vi "PLUXmereni.vi"() -> (1 "XY graph visual":cluster{dbl[], dbl[]}(graph))   [LabVIEW 2026]
uses:
  <userlib>/Status.ctl
  <vilib>/Analysis/3filter.llb/Butterworth Filter (DBL).vi
  <vilib>/measure/maspectr.llb/FFT Spectrum (Mag-Phase) for N Chan.vi
  <vilib>/Instr/_visa.llb/VISA Configure Serial Port (Instr).vi
  <vilib>/measure/NI_MAPro.lvlib
  <vilib>/Analysis/NI_AALBase.lvlib
panel:
  out "Array of signals":waveform(dbl)[](array[waveform])
  out "Spectrum":cluster{"f0":dbl, "df":dbl, "magnitude":dbl[]}[](graph)
  in  "EditCluster":T1={"Horní mezní frekvence"=0.45000000000000007, "Dolní mezní frekvence"=0.0, "filter type"=enum."Lowpass", "applyFilter"=FALSE, "removeFilter"=FALSE, "undoFIlter"=FALSE} {"Horní mezní frekvence" format="%0.2f"}
  out "Waveform Graph Edit":waveform(dbl)[](graph)
  out "Zobrazeni typu signalu":cluster{string, string}
  in  "Exit Button":bool
  out "NewVal":bool
  in  "MereniAZpracovaniSwitch":bool
  in  "Cluster":T2={"Zařízení"="", "Cesta k uloženému souboru"=path "", "Vzorkovací frekvence"=enum."1000", "Record Button"=FALSE, "Stop Button"=FALSE, "A1 signál"=enum."EMG", "A2 signál"=enum."EMG", "A3 signál"=enum."EMG", "A4 signál"=enum."EMG", "A5 signál"=enum."EMG", "A6 signál"=enum."EMG", "Pin s připojeným signálem"=enum."A1"}
  in  "DO 4":bool
  in  "DO 3":bool
  in  "DO 2":bool
  in  "DO 1":bool
  out "tdms file":refnum<k34>
  out "Ylabel and Plot name":cluster{string, string}
  out "Sample Rate Numeric":i32
  out "Consumer":i32
  out "producer":i32
  in  "error in (no error)":errorcluster
  out "Sync Stop":bool=TRUE
  # "Aplikace pro měření a zpracování dat na platformě PLUX BITalino"
  # "Spodní tlačítko bude jako switch mez iměřením a zpracováním                     tlačítka filtr, odstranit filtraci, undo"
  # "Hz"
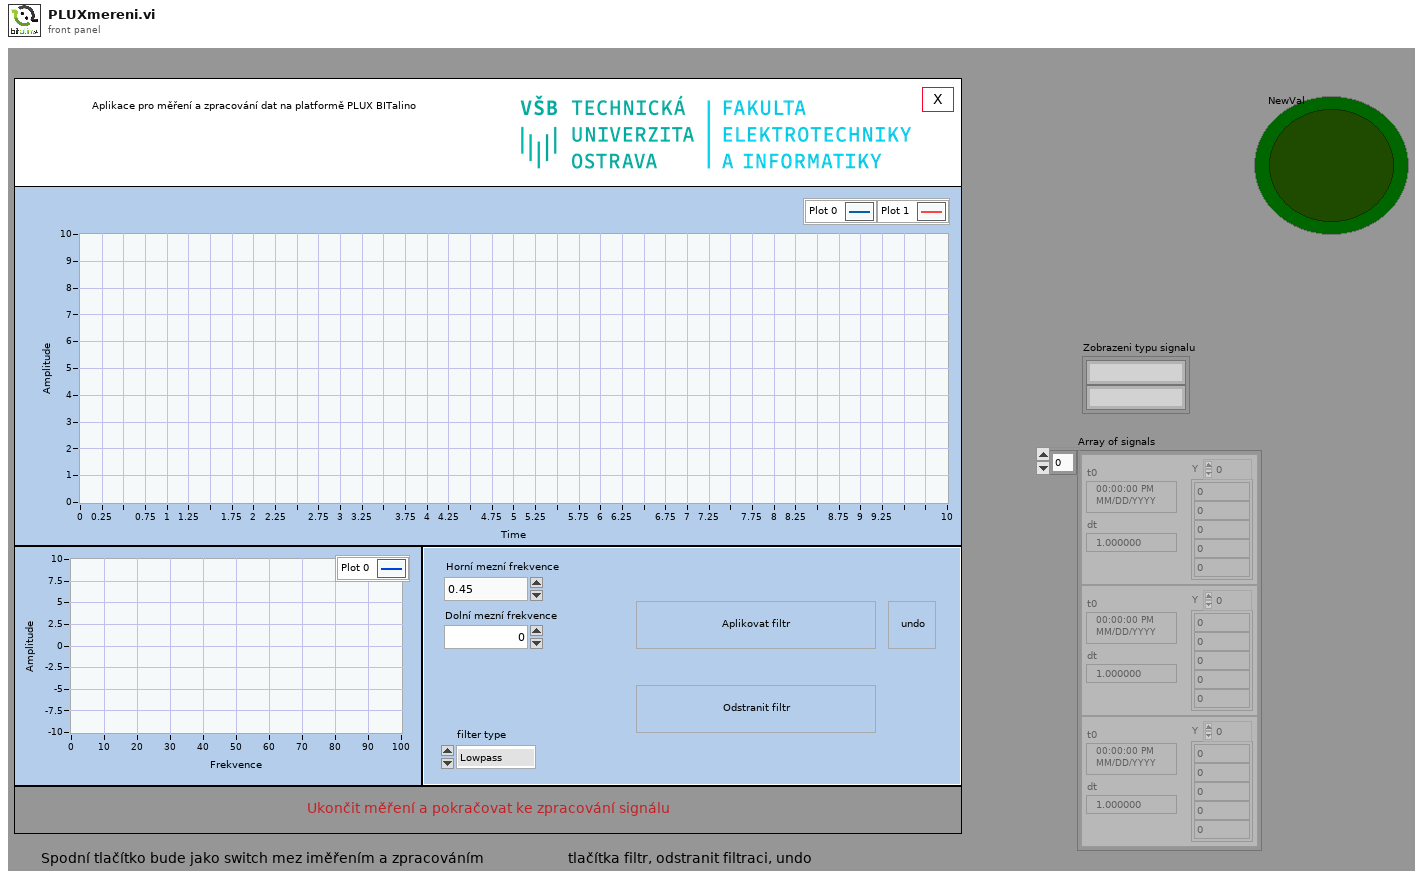
[diagram p1: front panel]
types:
  T1 = cluster{"Horní mezní frekvence":dbl, "Dolní mezní frekvence":dbl, "filter type":enum32{"Lowpass", "Highpass", "Bandpass", "Bandstop"}, "applyFilter":bool, "removeFilter":bool, "undoFIlter":bool}
  T2 = cluster{"Zařízení":refnum<visa-resource-name>, "Cesta k uloženému souboru":path, "Vzorkovací frekvence":enum16{"1", "10", "100", "1000"}, "Record Button":bool, "Stop Button":bool, "A1 signál":enum16{"EMG", "ECG", "EEG", "EDA", "ACC"}, "A2 signál":enum16{"EMG", "ECG", "EEG", "EDA", "ACC"}, "A3 signál":enum16{"EMG", "ECG", "EEG", "EDA", "ACC"}, "A4 signál":enum16{"EMG", "ECG", "EEG", "EDA", "ACC"}, "A5 signál":enum16{"EMG", "ECG", "EEG", "EDA", "ACC"}, "A6 signál":enum16{"EMG", "ECG", "EEG", "EDA", "ACC"}, "Pin s připojeným signálem":enum32{"A1", "A2", "A3", "A4", "A5", "A6"}}
  T3 = enum8{"Enabled", "Disabled", "Disabled and Grayed Out"}
  T4 = enum16{"open", "open or create", "create or replace", "create", "open (read-only)"}
  T5 = typedef "Status.ctl" = enum16{"Initialize", "Edit", "Standby", "Recording", "Exit"}
  T6 = enum32{"Lowpass", "Highpass", "Bandpass", "Bandstop"}
  T7 = cluster{"A1 signál":enum16{"EMG", "ECG", "EEG", "EDA", "ACC"}, "A2 signál":enum16{"EMG", "ECG", "EEG", "EDA", "ACC"}, "A3 signál":enum16{"EMG", "ECG", "EEG", "EDA", "ACC"}, "A4 signál":enum16{"EMG", "ECG", "EEG", "EDA", "ACC"}, "A5 signál":enum16{"EMG", "ECG", "EEG", "EDA", "ACC"}, "A6 signál":enum16{"EMG", "ECG", "EEG", "EDA", "ACC"}}
  T8 = cluster{"Result":dbl, "Result":dbl, "Result":dbl, "Result":dbl, "Result":dbl, "Result":dbl}
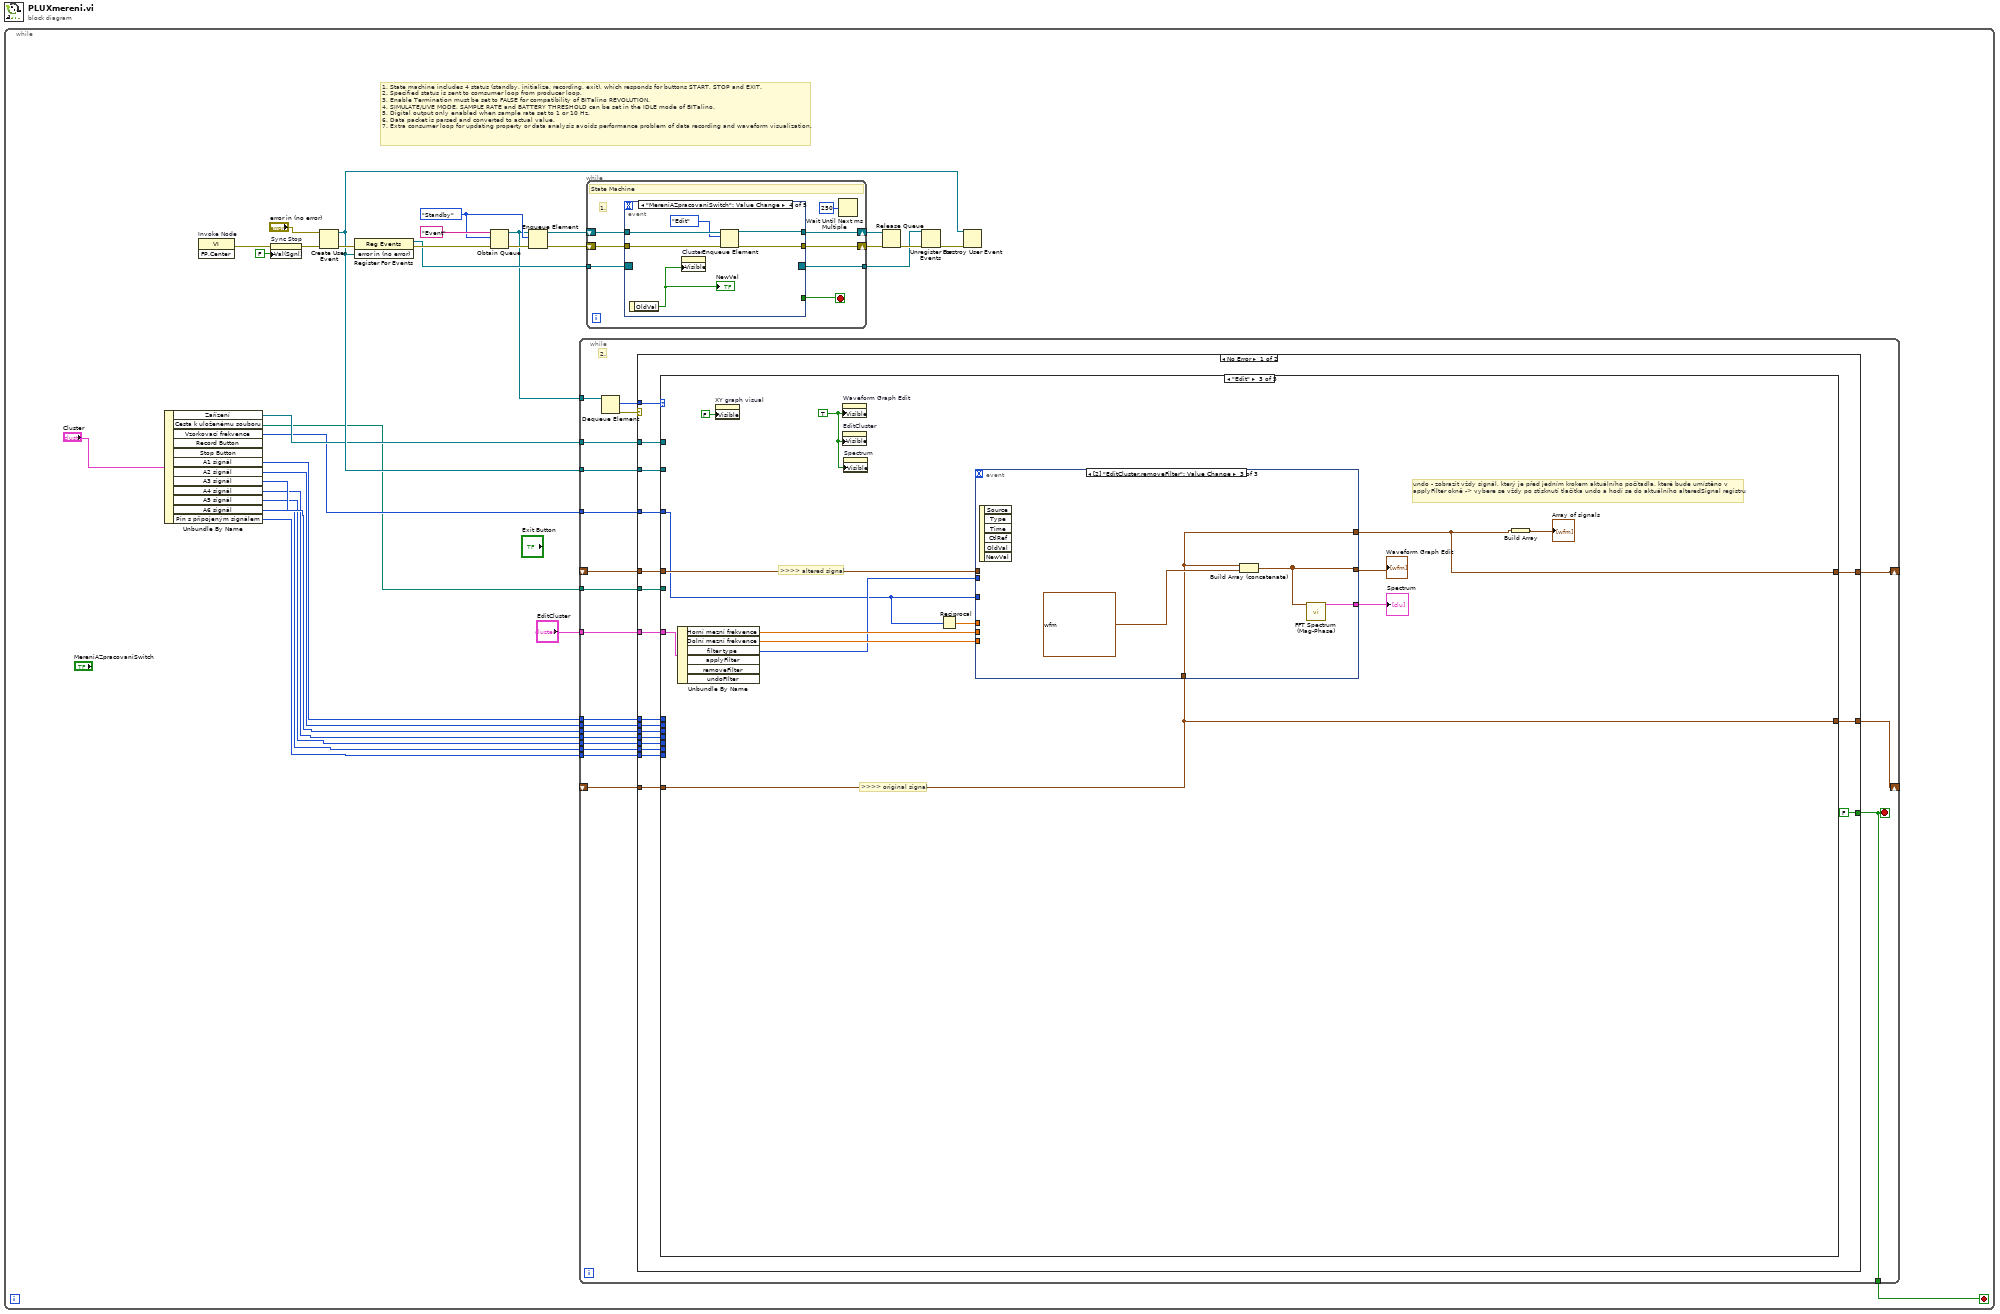
[diagram p0: block diagram]
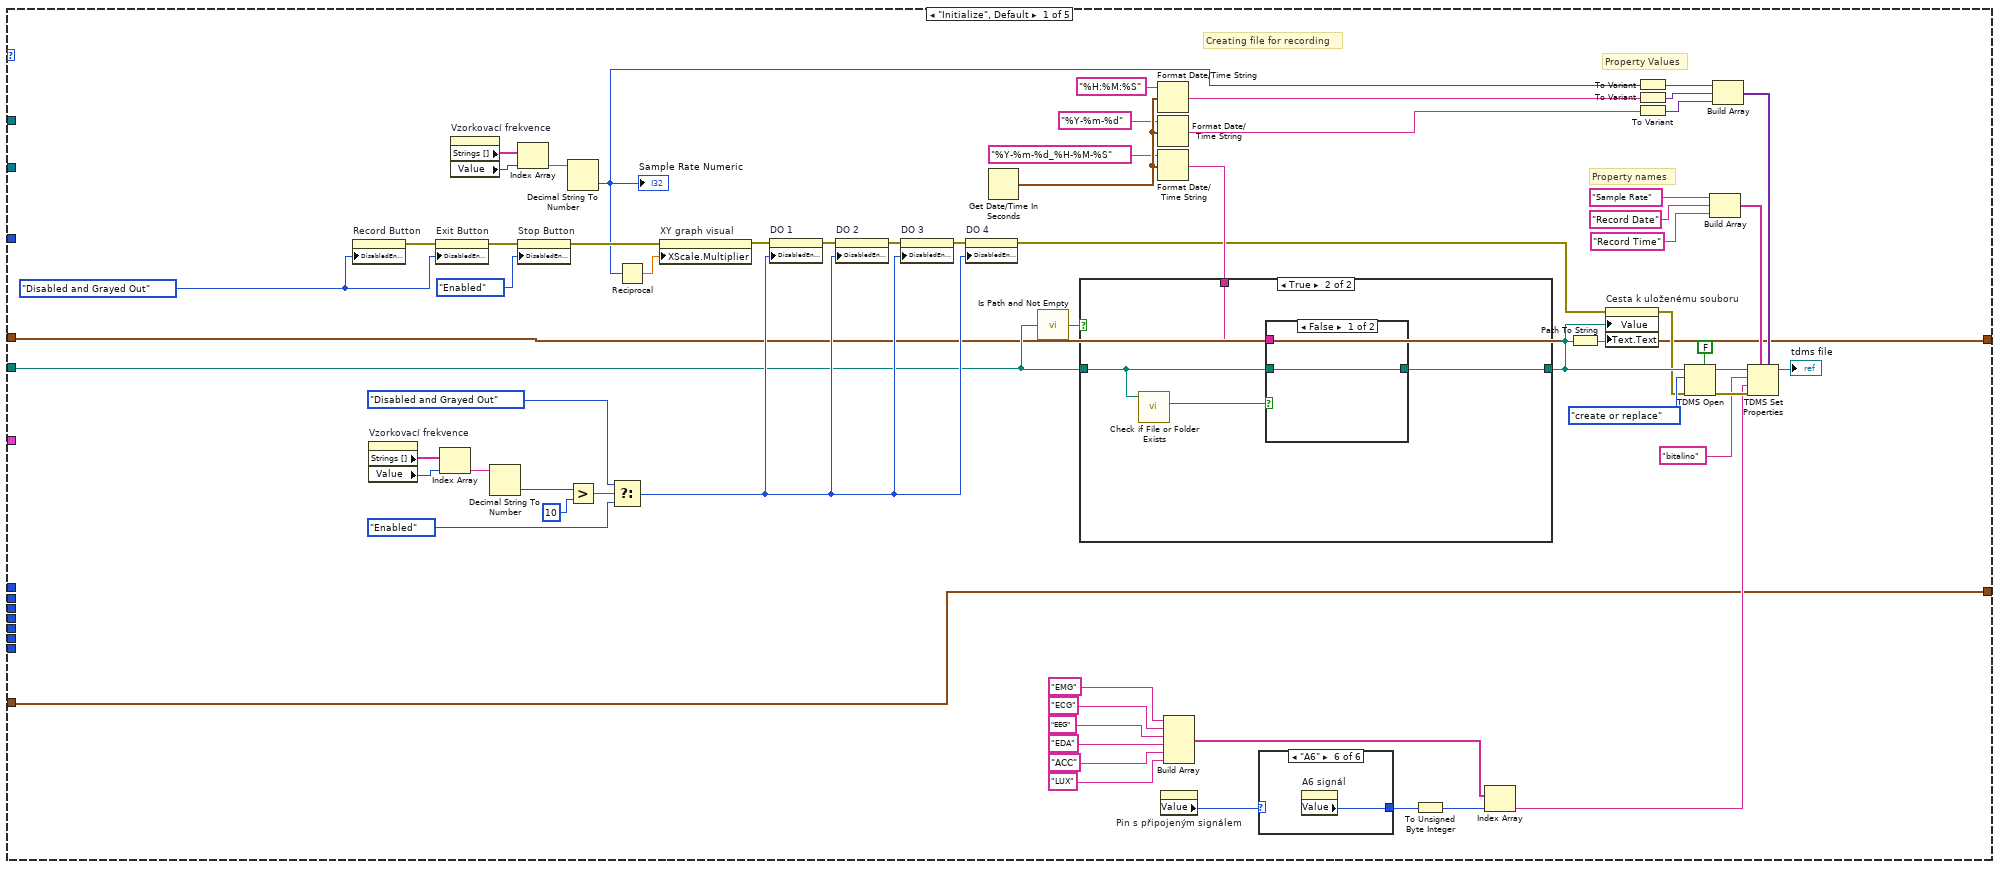
[diagram p2: hidden frame]
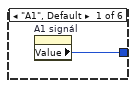
[diagram p3: hidden frame]
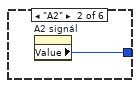
[diagram p4: hidden frame]
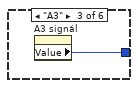
[diagram p5: hidden frame]
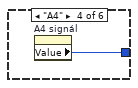
[diagram p6: hidden frame]
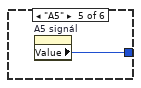
[diagram p7: hidden frame]
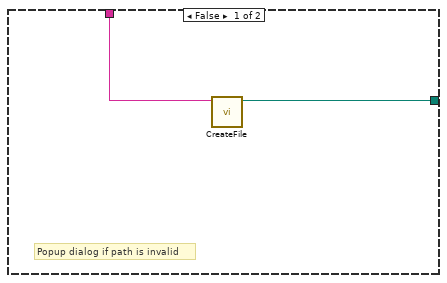
[diagram p8: hidden frame]
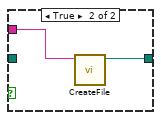
[diagram p9: hidden frame]
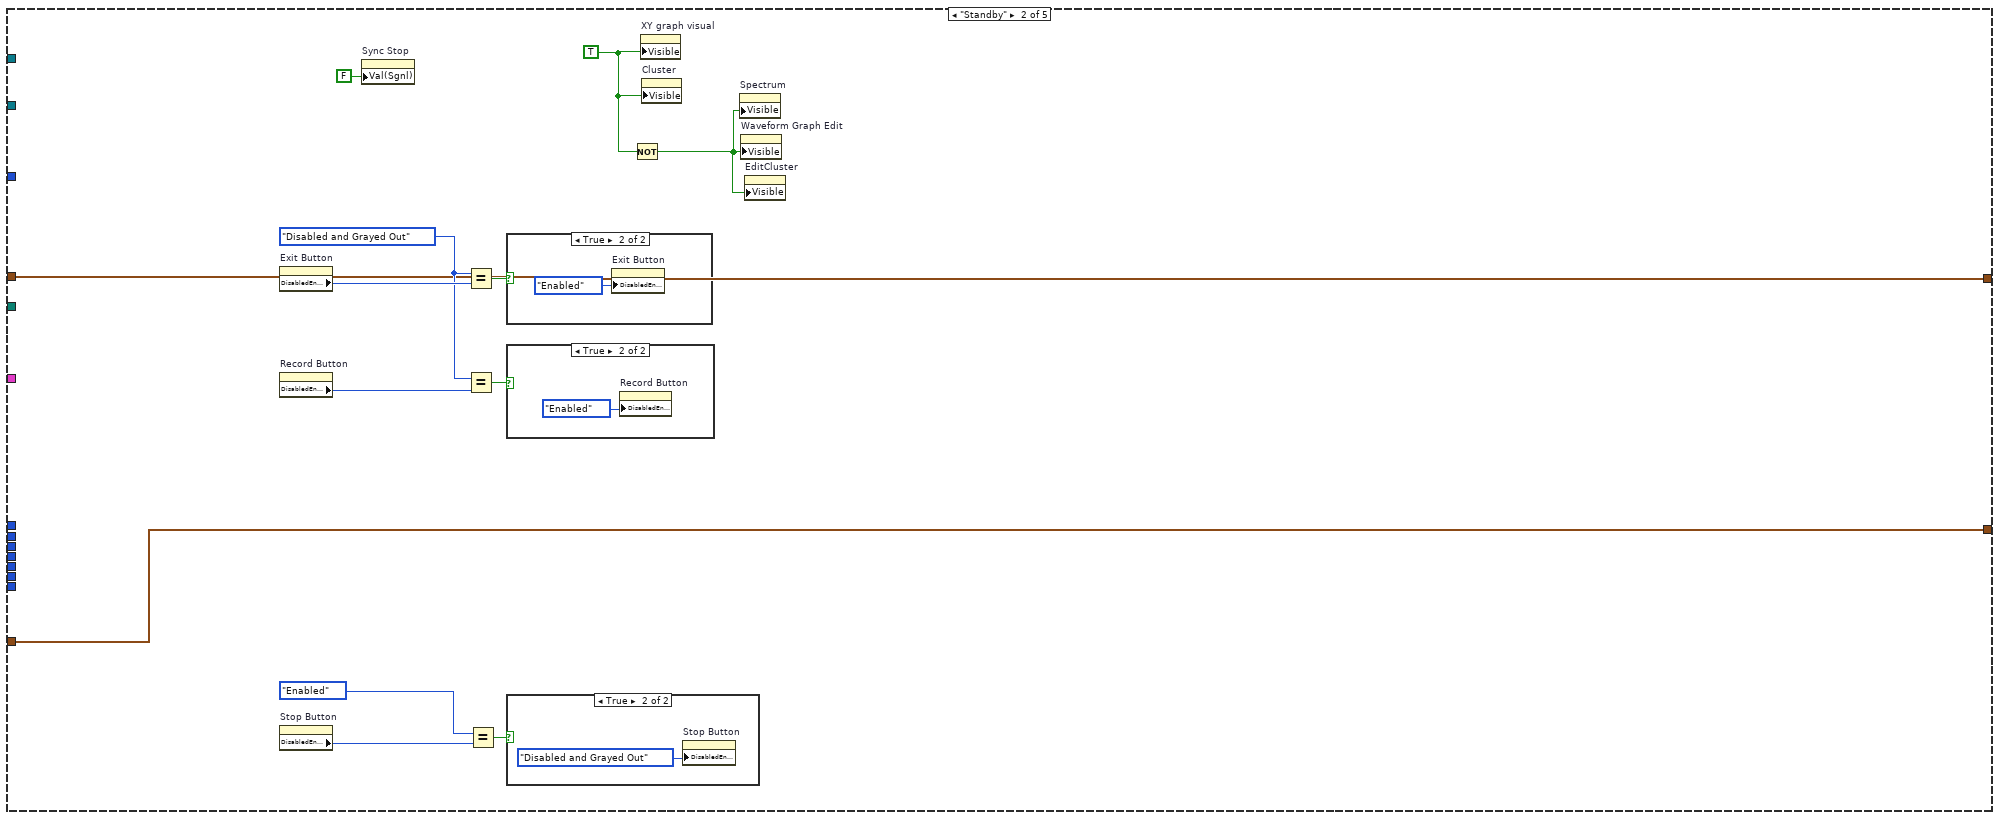
[diagram p10: hidden frame]
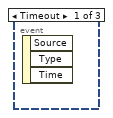
[diagram p14: hidden frame]
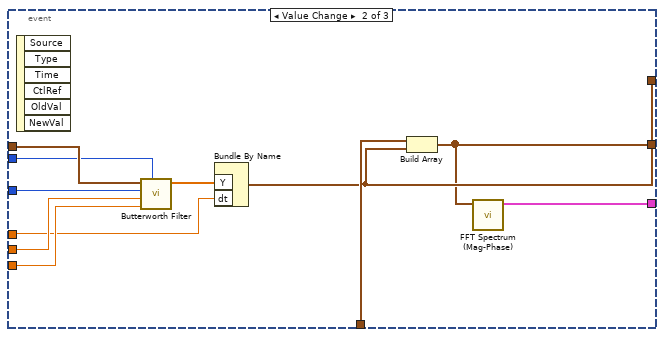
[diagram p15: hidden frame]
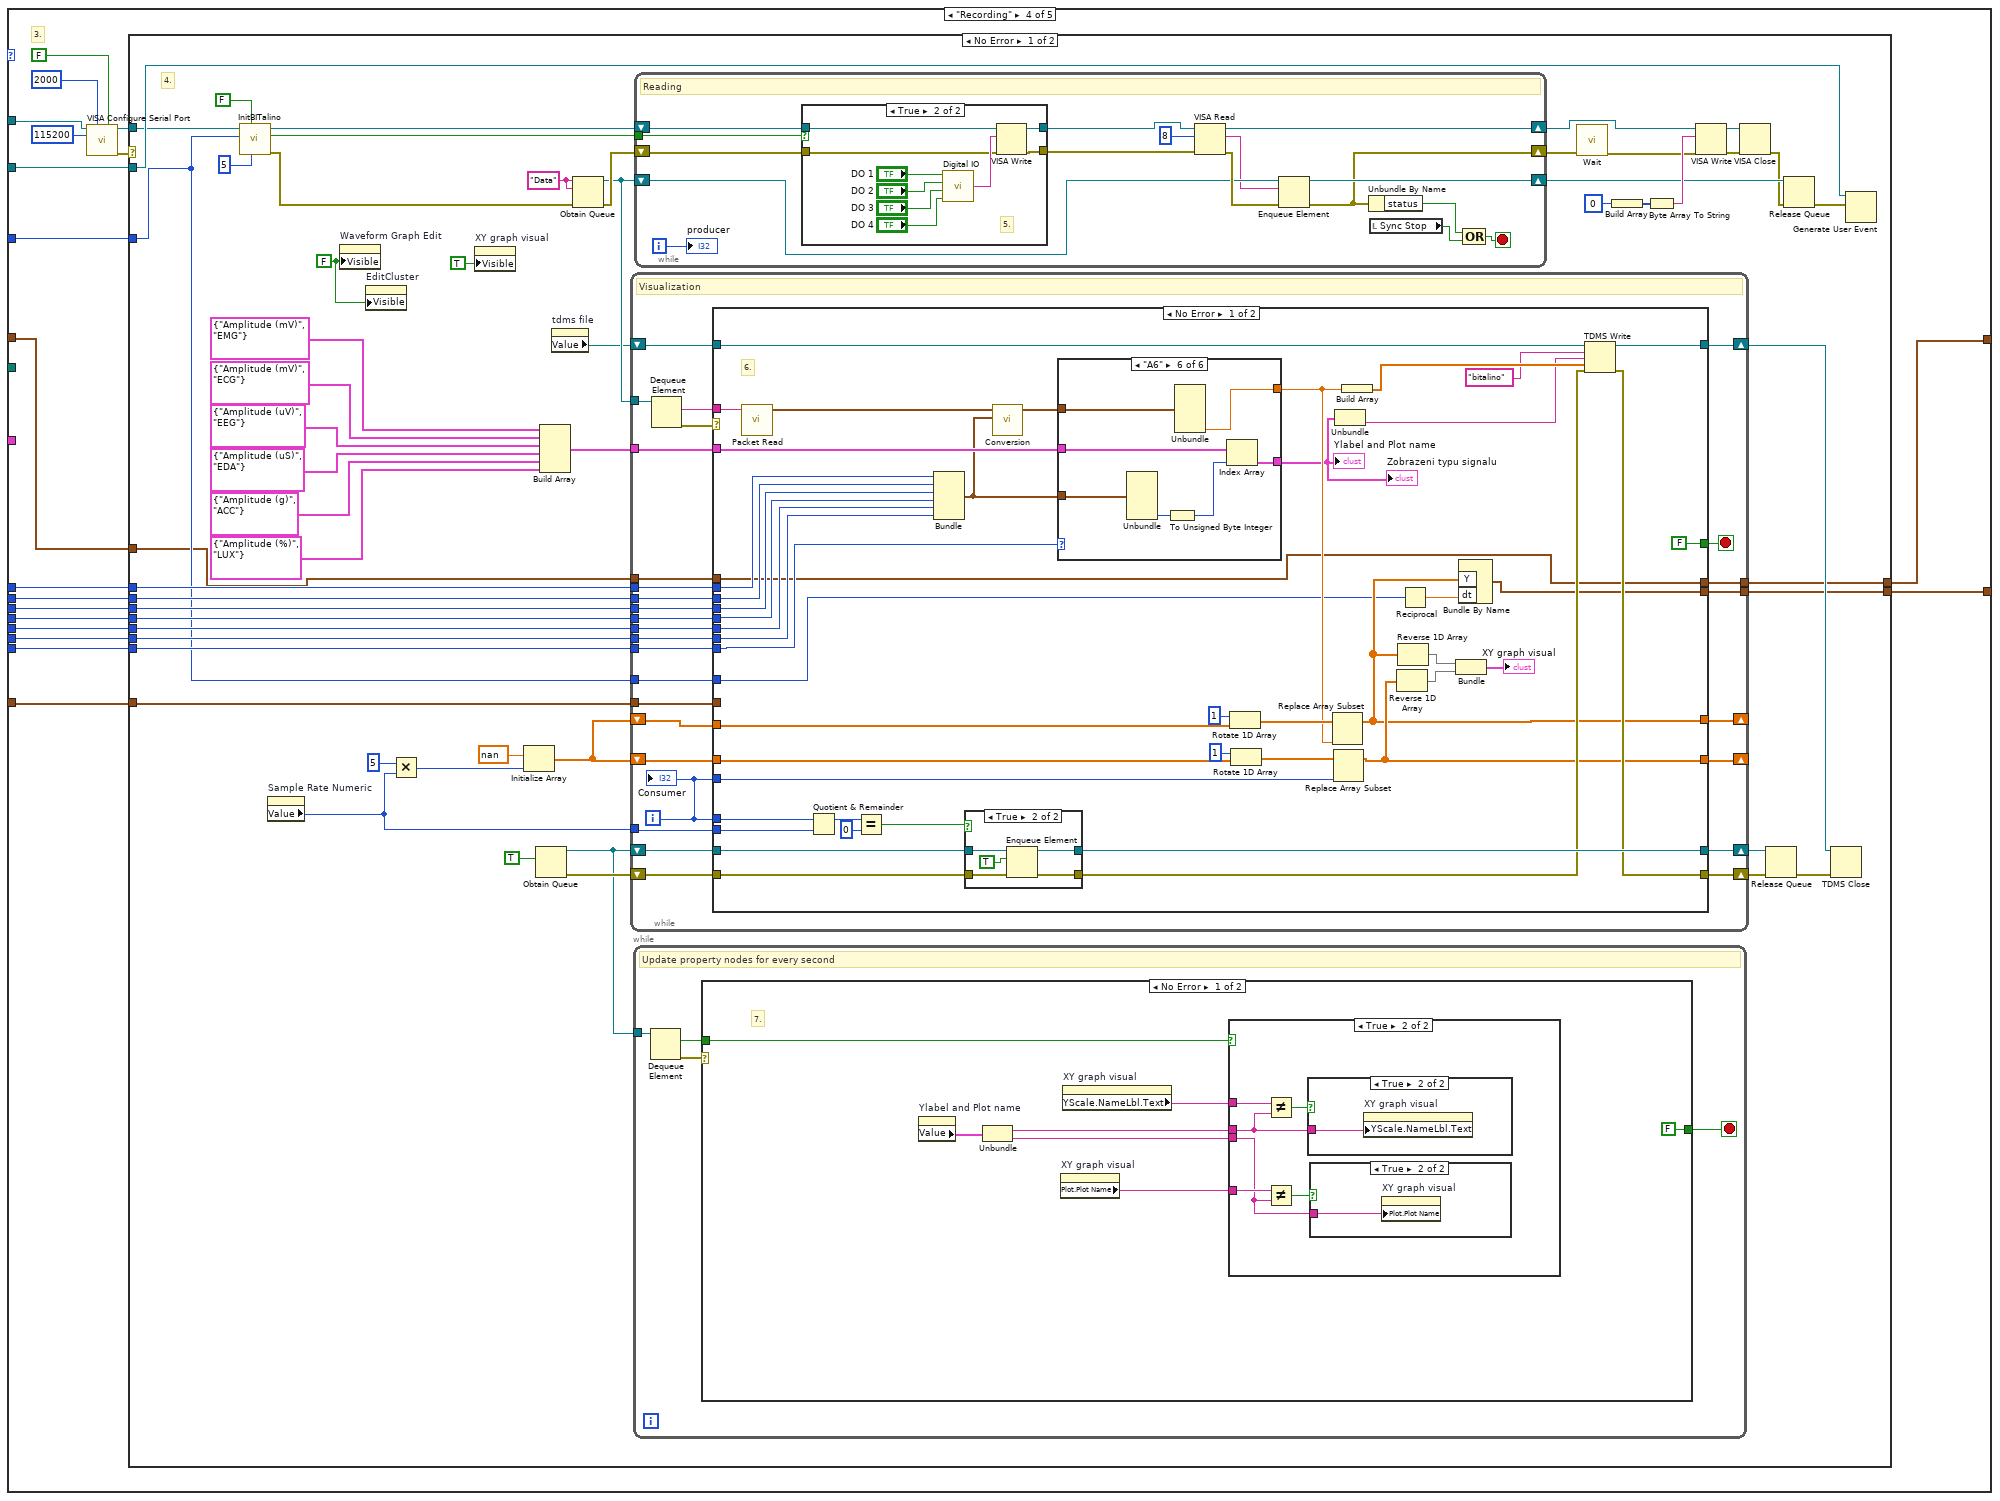
[diagram p16: hidden frame]
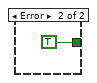
[diagram p20: hidden frame]
diagram:
  n1 = while {
    stop <- w3 stop-if-true
    w31 = Status."Standby" ("Enum")
    # "1. State machine includes 4 status (standby, initialize, recording, exit), which responds for buttons START, STOP and EXIT.\n2. Specified status is sent to comsumer loop from producer loop.\n3. Enable Termination must be set to FALSE for compatibility of BITalino REVOLUTION.\n4. SIMULATE/LIVE MODE, SAMPLE RATE and BATTERY THRESHOLD can be set in the IDLE mode of BITalino.\n5. Digital output only enabled when sample rate set to 1 or 10 Hz.\n6. Data packet is parsed and converted to actual value.\n7. Extra consumer loop for updating property or data analysis avoids performance problem of data recording and waveform visualization."
    n2 = Unbundle By Name("Cluster") -> ("Zařízení"=w13:refnum<visa-resource-name>, "Cesta k uloženému souboru"=w4:path, "Vzorkovací frekvence"=w12:enum16{"1", "10", "100", "1000"}, "A1 signál"=w11:enum16{"EMG", "ECG", "EEG", "EDA", "ACC"}, "A2 signál"=w10:enum16{"EMG", "ECG", "EEG", "EDA", "ACC"}, "A3 signál"=w9:enum16{"EMG", "ECG", "EEG", "EDA", "ACC"}, "A4 signál"=w8:enum16{"EMG", "ECG", "EEG", "EDA", "ACC"}, "A5 signál"=w7:enum16{"EMG", "ECG", "EEG", "EDA", "ACC"}, "A6 signál"=w6:enum16{"EMG", "ECG", "EEG", "EDA", "ACC"}, "Pin s připojeným signálem"=w5:enum32{"A1", "A2", "A3", "A4", "A5", "A6"})  [unwired: 2 out]
    n3 = invoke on="Invoke Node" class="VI" method="FP.Center"() -> (error out=w15:errorcluster)  [unwired: 3 in, 2 out]
    n4 = property on="Sync Stop" class="Bool (strict)"(error in=w15, "Val(Sgnl)"=FALSE ("Value (Signaling)")) -> (error out=w24:errorcluster)  [unwired: 1 in, 1 out]
    n5 = Create User Event(user event datatype="error in (no error)", error in=w24) -> (user event=w16:refnum<user-event>, error out=w23:errorcluster)
    n6 = register-events(error in=w23, w16) -> (reference out=w21:refnum<event-registration>, error out=w22:errorcluster)  [unwired: 1 in]
    n7 = Obtain Queue(name (unnamed)="Event", element data type=w31, error in (no error)=w22) -> (queue out=w14:refnum<queue>, error out=w27:errorcluster)  [unwired: 2 in, 1 out]
    n8 = Enqueue Element(queue=w14, element=w31, error in (no error)=w27) -> (queue out=w25:refnum<queue>, error out=w26:errorcluster)  [unwired: 1 in, 1 out]
    n9 = while {
      tunnel: w14 -> [w52]
      tunnel: w16 -> [w49]
      tunnel: w12 -> [w48]
      tunnel: [w47] -> w3
      tunnel: w13 -> [w46]
      tunnel: w11 -> [w45]
      tunnel: w10 -> [w44]
      tunnel: w9 -> [w43]
      tunnel: w8 -> [w42]
      tunnel: w7 -> [w41]
      tunnel: w6 -> [w40]
      tunnel: w5 -> [w39]
      tunnel: w4 -> [w38]
      shift-right: [w37] -> _
      shift-left: _ -> [w36]
      tunnel: "EditCluster" -> [w35]
      shift-right: [w34] -> _
      shift-left: _ -> [w33]
      stop <- w47 stop-if-true
      # "2."
      n10 = Dequeue Element(queue=w52) -> (element=w51:T5, error out=w50:errorcluster)  [unwired: 2 in, 2 out]
      n11 = case shown="No Error" w50 {
        tunnel: w51 -> [w67 _]
        tunnel: [FALSE TRUE] -> w47
        tunnel: w49 -> [w69 _]
        tunnel: w48 -> [w68 _]
        tunnel: w46 -> [w66 _]
        tunnel: w45 -> [w65 _]
        tunnel: w44 -> [w64 _]
        tunnel: w43 -> [w63 _]
        tunnel: w42 -> [w62 _]
        tunnel: w41 -> [w61 _]
        tunnel: w40 -> [w60 _]
        tunnel: w39 -> [w59 _]
        tunnel: w38 -> [w58 _]
        tunnel: [w57 w456] -> w37
        tunnel: w36 -> [w56 w456]
        tunnel: w35 -> [w55 _]
        tunnel: [w54 w455] -> w34
        tunnel: w33 -> [w53 w455]
        frame No Error {
          n12 = case shown="\"Edit\"" w67 {
            tunnel: w69 -> [_ _ _ w207 _]
            tunnel: w68 -> [_ _ w170 w206 _]
            tunnel: w66 -> [_ _ _ w205 _]
            tunnel: w65 -> [_ _ _ w204 _]
            tunnel: w64 -> [_ _ _ w203 _]
            tunnel: w63 -> [_ _ _ w202 _]
            tunnel: w62 -> [_ _ _ w201 _]
            tunnel: w61 -> [_ _ _ w200 _]
            tunnel: w60 -> [_ _ _ w199 _]
            tunnel: w59 -> [_ _ _ w198 _]
            tunnel: w58 -> [w73 _ _ _ _]
            tunnel: [w72 w152 w167 w197 w452] -> w57
            tunnel: w56 -> [w72 w152 w167 w196 w452]
            tunnel: w55 -> [_ _ w177 _ _]
            tunnel: [w71 w151 w166 w195 w451] -> w54
            tunnel: w53 -> [w71 w151 w175 w194 w451]
            frame "Initialize", Default {
              w101 = T3."Disabled and Grayed Out" ("Disabled")
              # "Creating file for recording"
              # "Property Values"
              # "Property names"
              n13 = property on="Record Button" class="Bool"("DisabledEnum"=w101) -> (error out=w133:errorcluster)  [unwired: 2 in, 1 out]
              n14 = property on="Vzorkovací frekvence" class="Enum (strict)"() -> ("Strings []"=w91:string[], "Value"=w90:enum16{"1", "10", "100", "1000"})  [unwired: 2 in, 2 out]
              n15 = property on="Exit Button" class="Bool"(error in=w133, "DisabledEnum"=w101) -> (error out=w131:errorcluster)  [unwired: 1 in, 1 out]
              n16 = Index Array "Index Array"(array=w91, index=w90) -> (element=w89:string)
              n17 = property on="Vzorkovací frekvence" class="Enum (strict)"() -> ("Strings []"=w130:string[], "Value"=w129:enum16{"1", "10", "100", "1000"})  [unwired: 2 in, 2 out]
              n18 = Decimal String To Number(string=w89) -> (number=w88:i32)  [unwired: 2 in, 1 out]
              n19 = Index Array(array=w130, index=w129) -> (element=w128:string)
              n20 = property on="Stop Button" class="Bool"(error in=w131, "DisabledEnum"=T3."Enabled" ("Disabled")) -> (error out=w127:errorcluster)  [unwired: 1 in, 1 out]
              n21 = Decimal String To Number(string=w128) -> (number=w100:i32)  [unwired: 2 in, 1 out]
              "Sample Rate Numeric" <- w100
              n22 = Greater?(x=w88, y=10) -> (0:w96:bool)
              n23 = Select(t=T3."Disabled and Grayed Out" ("Disabled"), s=w96, f=T3."Enabled" ("Disabled")) -> (s? t:f=w99:T3)
              n24 = Reciprocal(x=w100) -> (1/x=w126:dbl)
              n25 = property on="XY graph visual" class="XYGraph (strict)"(error in=w127, "XScale.Multiplier"=w126) -> (error out=w87:errorcluster)  [unwired: 1 in, 1 out]
              n26 = property on="DO 1" class="Bool (strict)"(error in=w87, "DisabledEnum"=w99) -> (error out=w94:errorcluster)  [unwired: 1 in, 1 out]
              n27 = property on="DO 2" class="Bool (strict)"(error in=w94, "DisabledEnum"=w99) -> (error out=w93:errorcluster)  [unwired: 1 in, 1 out]
              n28 = property on="DO 3" class="Bool (strict)"(error in=w93, "DisabledEnum"=w99) -> (error out=w92:errorcluster)  [unwired: 1 in, 1 out]
              n29 = property on="DO 4" class="Bool (strict)"(error in=w92, "DisabledEnum"=w99) -> (error out=w86:errorcluster)  [unwired: 1 in, 1 out]
              n30 = Get Date/Time In Seconds() -> (seconds since 1Jan1904=w116:timestamp)
              n31 = call <vilib>:"Is Path and Not Empty.vi"("path"=w73) -> ("Is Path and Not Empty?"=w108:bool)  [unwired: 4 in]
              n32 = Format Date/Time String(time format string (%c)="%H:%M:%S", seconds (now)=w116) -> (date/time string=w121:string)  [unwired: 1 in]
              n33 = Format Date/Time String(time format string (%c)="%Y-%m-%d", seconds (now)=w116) -> (date/time string=w122:string)  [unwired: 1 in]
              n34 = Format Date/Time String(time format string (%c)="%Y-%m-%d_%H-%M-%S", seconds (now)=w116) -> (date/time string=w112:string)  [unwired: 1 in]
              n35 = case shown="True" w108 {
                tunnel: [w140 w143] -> w105
                tunnel: w73 -> [_ w142]
                tunnel: w112 -> [w141 w144]
                frame False {
                  # "Popup dialog if path is invalid"
                  n36 = call <userlib>:"CreateFile.vi"("date/time string"=w141) -> ("appended path"=w140:path)  [unwired: 10 in]
                }
                frame True {
                  n37 = call <vilib>:"Check if File or Folder Exists.vi"("path"=w142) -> ("file or folder exists?"=w145:bool)  [unwired: 8 in, 2 out]
                  n38 = case shown="False" w145 {
                    tunnel: w144 -> [_ w148]
                    tunnel: [w146 w147] -> w143
                    tunnel: w142 -> [w146 _]
                    frame False {
                    }
                    frame True {
                      n39 = call <userlib>:"CreateFile.vi"("date/time string"=w148) -> ("appended path"=w147:path)  [unwired: 10 in]
                    }
                  }
                }
              }
              n40 = property on="Pin s připojeným signálem" class="RadioBtnsControl (strict)"() -> ("Value"=w84:enum32{"A1", "A2", "A3", "A4", "A5", "A6"})  [unwired: 2 in, 2 out]
              n41 = Build Array("EMG", "ECG", "EEG", "EDA", "ACC", "LUX") -> (w75:string[])
              n42 = case shown="\"A6\"" w84 {
                tunnel: [w134 w135 w136 w137 w138 w139] -> w77
                frame "A1", Default {
                  n43 = property on="A1 signál" class="Enum (strict)"() -> ("Value"=w134:enum16{"EMG", "ECG", "EEG", "EDA", "ACC"})  [unwired: 2 in, 2 out]
                }
                frame "A2" {
                  n44 = property on="A2 signál" class="Enum (strict)"() -> ("Value"=w135:enum16{"EMG", "ECG", "EEG", "EDA", "ACC"})  [unwired: 2 in, 2 out]
                }
                frame "A3" {
                  n45 = property on="A3 signál" class="Enum (strict)"() -> ("Value"=w136:enum16{"EMG", "ECG", "EEG", "EDA", "ACC"})  [unwired: 2 in, 2 out]
                }
                frame "A4" {
                  n46 = property on="A4 signál" class="Enum (strict)"() -> ("Value"=w137:enum16{"EMG", "ECG", "EEG", "EDA", "ACC"})  [unwired: 2 in, 2 out]
                }
                frame "A5" {
                  n47 = property on="A5 signál" class="Enum (strict)"() -> ("Value"=w138:enum16{"EMG", "ECG", "EEG", "EDA", "ACC"})  [unwired: 2 in, 2 out]
                }
                frame "A6" {
                  n48 = property on="A6 signál" class="Enum (strict)"() -> ("Value"=w139:enum16{"EMG", "ECG", "EEG", "EDA", "ACC"})  [unwired: 2 in, 2 out]
                }
              }
              n49 = To Unsigned Byte Integer(number=w77) -> (unsigned 8bit integer=w76:u8)
              n50 = Index Array(array=w75, index=w76) -> (element=w74:string)
              n51 = Path To String(path=w105) -> (string=w106:string)
              n52 = property on="Cesta k uloženému souboru" class="Path"(error in=w86, "Value"=w105, "Text.Text"=w106) -> (error out=w104:errorcluster)  [unwired: 1 in, 1 out]
              n53 = To Variant(anything=w100) -> (Variant=w120:variant)
              n54 = To Variant(anything=w121) -> (Variant=w123:variant)
              n55 = To Variant(anything=w122) -> (Variant=w124:variant)
              n56 = TDMS Open(5:FALSE ("create index file? (T)"), 8:w104, 10:T4."create or replace" ("operation (0:open)"), 11:w105) -> (0:w111:errorcluster, 3:w110:refnum<k34>)  [unwired: 3 in]
              n57 = Build Array("Sample Rate", "Record Date", "Record Time") -> (w119:string[])
              n58 = Build Array(w120, w123, w124) -> (w125:variant[])
              n59 = TDMS Set Properties(5:w125, 7:w119, 8:w111, 9:w74, 10:"bitalino", 11:w110) -> (3:→"tdms file":refnum<k34>)  [unwired: 3 out]
            }
            frame "Standby" {
              w150 = TRUE ("Visible")
              w153 = T3."Disabled and Grayed Out" ("Disabled")
              n60 = property on="Exit Button" class="Bool"() -> ("DisabledEnum"=w160:T3)  [unwired: 2 in, 2 out]
              n61 = property on="Record Button" class="Bool"() -> ("DisabledEnum"=w158:T3)  [unwired: 2 in, 2 out]
              n62 = property on="Stop Button" class="Bool"() -> ("DisabledEnum"=w155:T3)  [unwired: 2 in, 2 out]
              n63 = property on="Sync Stop" class="Bool (strict)"("Val(Sgnl)"=FALSE ("Value (Signaling)")) -> ()  [unwired: 2 in, 2 out]
              n64 = Equal?(x=w153, y=w160) -> (x = y?=w159:bool)
              n65 = Equal?(x=w153, y=w158) -> (x = y?=w157:bool)
              n66 = Equal?(x=T3."Enabled" ("Disabled"), y=w155) -> (x = y?=w154:bool)
              n67 = case shown="True" w159 {
                frame False {
                }
                frame True {
                  n68 = property on="Exit Button" class="Bool"("DisabledEnum"=T3."Enabled" ("Disabled")) -> ()  [unwired: 2 in, 2 out]
                }
              }
              n69 = case shown="True" w157 {
                frame False {
                }
                frame True {
                  n70 = property on="Record Button" class="Bool"("DisabledEnum"=T3."Enabled" ("Disabled")) -> ()  [unwired: 2 in, 2 out]
                }
              }
              n71 = case shown="True" w154 {
                frame False {
                }
                frame True {
                  n72 = property on="Stop Button" class="Bool"("DisabledEnum"=T3."Disabled and Grayed Out" ("Disabled")) -> ()  [unwired: 2 in, 2 out]
                }
              }
              n73 = Not(x=w150) -> (.not. x?=w149:bool)
              n74 = property on="XY graph visual" class="XYGraph (strict)"("Visible"=w150) -> ()  [unwired: 2 in, 2 out]
              n75 = property on="Cluster" class="Clust"("Visible"=w150) -> ()  [unwired: 2 in, 2 out]
              n76 = property on="Spectrum" class="WFGraph (strict)"("Visible"=w149) -> ()  [unwired: 2 in, 2 out]
              n77 = property on="Waveform Graph Edit" class="WFGraph (strict)"("Visible"=w149) -> ()  [unwired: 2 in, 2 out]
              n78 = property on="EditCluster" class="Clust"("Visible"=w149) -> ()  [unwired: 2 in, 2 out]
            }
            frame "Edit" {
              w176 = TRUE ("Visible")
              # "undo - zobrazit vždy signál, který je před jedním krokem aktuálního počítadla, které bude umístěno v \napplyFilter okně -> vybere se vždy po stisknutí tlačítka undo a hodí se do aktuálního alteredSignal registru"
              # ">>>> altered signal"
              # ">>>> original signal"
              n79 = Unbundle By Name(w177) -> ("Horní mezní frekvence"=w173:dbl, "Dolní mezní frekvence"=w172:dbl, "filter type"=w171:T6)  [unwired: 3 out]
              n80 = property on="XY graph visual" class="XYGraph (strict)"("Visible"=FALSE) -> ()  [unwired: 2 in, 2 out]
              n81 = property on="Waveform Graph Edit" class="WFGraph (strict)"("Visible"=w176) -> ()  [unwired: 2 in, 2 out]
              n82 = property on="EditCluster" class="Clust"("Visible"=w176) -> ()  [unwired: 2 in, 2 out]
              n83 = property on="Spectrum" class="WFGraph (strict)"("Visible"=w176) -> ()  [unwired: 2 in, 2 out]
              n84 = Reciprocal(x=w170) -> (1/x=w174:dbl)
              n85 = event shown="[2] \"EditCluster.removeFilter\": Value Change" {
                selector: _ -> [_ _ _]
                dyn-events: _ -> [_ _ _]
                timeout: _ -> [_ _ _]
                tunnel: w167 -> [_ w188 w190]
                tunnel: [_ w187 w190] -> w166
                tunnel: w175 -> [_ w186 _]
                tunnel: w174 -> [_ w182 _]
                tunnel: w173 -> [_ w185 _]
                tunnel: w172 -> [_ w184 _]
                tunnel: w171 -> [_ w183 _]
                tunnel: w170 -> [_ w181 _]
                tunnel: [_ w180 w191] -> w169
                tunnel: [_ w179 w192] -> w168
                event Timeout {
                  n86 = event-data() -> ()  [unwired: 1 in, 3 out]
                }
                event "EditCluster.applyFilter": Value Change {
                  n87 = event-data() -> ()  [unwired: 1 in, 6 out]
                  n88 = call-poly <vilib>:"Butterworth Filter.vi"("filter type"=w183, "low cutoff freq: fl"=w184, "high cutoff freq: fh"=w185, "sampling freq: fs"=w181, "X"=w186) -> ("Filtered X"=w189:dbl[])  [unwired: 3 in, 1 out]
                  n89 = Bundle By Name("Y"=w189, "dt"=w182) -> (w187:waveform(dbl))  [unwired: 1 in]
                  n90 = Build Array(w188, w187) -> (w180:waveform(dbl)[])
                  n91 = call-poly <vilib>:"FFT Spectrum (Mag-Phase).vi"("time signals"=w180) -> ("magnitudes"=w179:cluster{"f0":dbl, "df":dbl, "magnitude":dbl[]}[])  [unwired: 6 in, 4 out]
                }
                event "EditCluster.removeFilter": Value Change {
                  n92 = event-data() -> ()  [unwired: 1 in, 6 out]
                  n93 = Build Array (concatenate)(w190, waveform(dbl)[] [{"t0"=timestamp(-3600 s since 1904-01-01), "dt"=0.0, "Y"=[0.0]}] ("array")) -> (w191:waveform(dbl)[])
                  n94 = call-poly <vilib>:"FFT Spectrum (Mag-Phase).vi"("time signals"=w191) -> ("magnitudes"=w192:cluster{"f0":dbl, "df":dbl, "magnitude":dbl[]}[])  [unwired: 6 in, 4 out]
                }
              }
              "Waveform Graph Edit" <- w169
              "Spectrum" <- w168
              n95 = Build Array(w166) -> (→"Array of signals":waveform(dbl)[])
            }
            frame "Recording" {
              # "3."
              n96 = call-poly "VISA Configure Serial Port"("VISA resource name"=w205, "timeout (10sec)"=u32 2000, "Enable Termination\nChar (T)"=FALSE ("Enable Termination\nChar (T)"), "baud rate (9600)"=u32 115200) -> ("VISA resource name out"=w210:refnum<visa-resource-name>, "error out"=w209:errorcluster)  [unwired: 10 in]
              n97 = case shown="No Error" w209 {
                selector: w209 -> [_ w449]
                tunnel: w210 -> [w252 _]
                tunnel: w207 -> [w254 w450]
                tunnel: w206 -> [w219 _]
                tunnel: w204 -> [w228 _]
                tunnel: w203 -> [w227 _]
                tunnel: w202 -> [w226 _]
                tunnel: w201 -> [w225 _]
                tunnel: w200 -> [w224 _]
                tunnel: w199 -> [w223 _]
                tunnel: w198 -> [w222 _]
                tunnel: [w218 w448] -> w197
                tunnel: w196 -> [w216 w448]
                tunnel: [w215 w447] -> w195
                tunnel: w194 -> [w214 w447]
                frame No Error {
                  w213 = FALSE ("Visible")
                  w262 = "Data"
                  # "4."
                  n98 = call <userlib>:"InitBITalino.vi"("Battery \nThreshold (%)"=u8 5 ("Battery \nThreshold (%)"), "MODE"=FALSE, "Sample Rate"=w219, "BITalino"=w252) -> ("error out"=w230:errorcluster, "Digital Output"=w231:bool, "VISA out"=w232:refnum<visa-resource-name>)  [unwired: 5 in]
                  n99 = property on="Sample Rate Numeric" class="DigNum (strict)"() -> ("Value"=w246:i32)  [unwired: 2 in, 2 out]
                  n100 = property on="Waveform Graph Edit" class="WFGraph (strict)"("Visible"=w213) -> ()  [unwired: 2 in, 2 out]
                  n101 = property on="EditCluster" class="Clust"("Visible"=w213) -> ()  [unwired: 2 in, 2 out]
                  n102 = Multiply(x=5, y=w246) -> (x*y=w244:i32)
                  n103 = property on="XY graph visual" class="XYGraph (strict)"("Visible"=TRUE) -> ()  [unwired: 2 in, 2 out]
                  n104 = Initialize Array(nan ("element"), w244) -> (w243:dbl[])
                  n105 = Obtain Queue(element data type=TRUE) -> (queue out=w249:refnum<queue>, error out=w251:errorcluster)  [unwired: 4 in, 1 out]
                  n106 = Build Array(cluster{string, string} {"Amplitude (mV)", "EMG"}, cluster{string, string} {"Amplitude (mV)", "ECG"}, cluster{string, string} {"Amplitude (uV)", "EEG"}, cluster{string, string} {"Amplitude (uS)", "EDA"}, cluster{string, string} {"Amplitude (g)", "ACC"}, cluster{string, string} {"Amplitude (%)", "LUX"}) -> (w236:cluster{string, string}[])
                  n107 = property on="tdms file" class="Ref (strict)"() -> ("Value"=w235:refnum<k34>)  [unwired: 2 in, 2 out]
                  n108 = Obtain Queue(name (unnamed)=w262, element data type=w262, error in (no error)=w230) -> (queue out=w263:refnum<queue>, error out=w264:errorcluster)  [unwired: 2 in, 1 out]
                  n109 = while {
                    tunnel: w263 -> [w316]
                    shift-right: [w311] -> _
                    shift-left: w243 -> [w312]
                    tunnel: w246 -> [w310]
                    shift-right: [w307] -> w248
                    shift-left: w249 -> [w309]
                    shift-right: [w306] -> w247
                    shift-left: w251 -> [w308]
                    shift-right: [w303] -> _
                    shift-left: w243 -> [w305]
                    tunnel: w236 -> [w302]
                    shift-right: [w300] -> w233
                    shift-left: w235 -> [w301]
                    tunnel: w228 -> [w299]
                    tunnel: w227 -> [w298]
                    tunnel: w226 -> [w297]
                    tunnel: w225 -> [w296]
                    tunnel: w224 -> [w295]
                    tunnel: w223 -> [w294]
                    tunnel: w222 -> [w293]
                    tunnel: w219 -> [w292]
                    tunnel: [w291] -> w218
                    tunnel: w216 -> [w290]
                    tunnel: [w289] -> w215
                    tunnel: w214 -> [w288]
                    i -> [w304]
                    stop <- w314 stop-if-true
                    # "Visualization"
                    n110 = Dequeue Element(queue=w316) -> (element=w313:string, error out=w315:errorcluster)  [unwired: 2 in, 2 out]
                    n111 = case shown="No Error" w315 {
                      tunnel: [FALSE TRUE] -> w314
                      tunnel: w313 -> [w337 _]
                      tunnel: w312 -> [w350 w418]
                      tunnel: [w321 w418] -> w311
                      tunnel: w310 -> [w351 _]
                      tunnel: w304 -> [w356 _]
                      tunnel: w309 -> [w359 w417]
                      tunnel: w308 -> [w358 w416]
                      tunnel: [w357 w417] -> w307
                      tunnel: [w338 w416] -> w306
                      tunnel: w305 -> [w347 w415]
                      tunnel: w304 -> [w346 _]
                      tunnel: [w326 w415] -> w303
                      tunnel: w302 -> [w345 _]
                      tunnel: w301 -> [w343 w414]
                      tunnel: [w342 w414] -> w300
                      tunnel: w299 -> [w333 _]
                      tunnel: w298 -> [w332 _]
                      tunnel: w297 -> [w331 _]
                      tunnel: w296 -> [w330 _]
                      tunnel: w295 -> [w329 _]
                      tunnel: w294 -> [w328 _]
                      tunnel: w293 -> [w327 _]
                      tunnel: w292 -> [w319 _]
                      tunnel: [w318 w413] -> w291
                      tunnel: w290 -> [_ w413]
                      tunnel: [w317 w412] -> w289
                      tunnel: w288 -> [w317 w412]
                      frame No Error {
                        # "6."
                        n112 = call <userlib>:"Packet Read.vi"("Packets"=w337) -> ("Analog Channels"=w336:cluster{u16, u16, u16, u16, u16, u16})  [unwired: 7 in, 3 out]
                        n113 = Quotient & Remainder(x=w356, y=w351) -> (x-y*floor(x/y)=w355:i32)  [unwired: 1 out]
                        n114 = Equal?(x=w355, y=0) -> (x = y?=w353:bool)
                        n115 = Bundle "Bundle"("A1 signál"=w333, "A2 signál"=w332, "A3 signál"=w331, "A4 signál"=w330, "A5 signál"=w329, "A6 signál"=w328) -> (w344:T7)  [unwired: 1 in]
                        n116 = case shown="True" w353 {
                          tunnel: w359 -> [w364 w369]
                          tunnel: w358 -> [w363 w368]
                          tunnel: [w364 w367] -> w357
                          tunnel: [w363 w366] -> w341
                          frame False {
                          }
                          frame True {
                            n117 = Enqueue Element(queue=w369, element=TRUE, error in (no error)=w368) -> (queue out=w367:refnum<queue>, error out=w366:errorcluster)  [unwired: 1 in, 1 out]
                          }
                        }
                        n118 = call <userlib>:"Conversion.vi"("Sensor Type"=w344, "Analog Channels"=w336) -> ("Converted Values"=w361:T8)  [unwired: 8 in, 1 out]
                        n119 = case shown="\"A6\"" w327 {
                          tunnel: w361 -> [w376 w383 w390 w397 w404 w411]
                          tunnel: [w375 w382 w389 w396 w403 w410] -> w340
                          tunnel: w345 -> [w371 w378 w385 w393 w399 w407]
                          tunnel: w344 -> [w374 w380 w387 w394 w401 w408]
                          tunnel: [w370 w377 w386 w392 w400 w406] -> w323
                          frame "A1", Default {
                            n120 = Unbundle(w374) -> ("A1 signál"=w372:enum16{"EMG", "ECG", "EEG", "EDA", "ACC"})  [unwired: 5 out]
                            n121 = To Unsigned Byte Integer(number=w372) -> (unsigned 8bit integer=w373:u8)
                            n122 = Unbundle(w376) -> ("Result"=w375:dbl)  [unwired: 5 out]
                            n123 = Index Array(array=w371, index=w373) -> (element=w370:cluster{string, string})
                          }
                          frame "A2" {
                            n124 = Unbundle(w380) -> ("A2 signál"=w379:enum16{"EMG", "ECG", "EEG", "EDA", "ACC"})  [unwired: 5 out]
                            n125 = To Unsigned Byte Integer(number=w379) -> (unsigned 8bit integer=w381:u8)
                            n126 = Unbundle(w383) -> ("Result"=w382:dbl)  [unwired: 5 out]
                            n127 = Index Array(array=w378, index=w381) -> (element=w377:cluster{string, string})
                          }
                          frame "A3" {
                            n128 = Unbundle(w387) -> ("A3 signál"=w384:enum16{"EMG", "ECG", "EEG", "EDA", "ACC"})  [unwired: 5 out]
                            n129 = To Unsigned Byte Integer(number=w384) -> (unsigned 8bit integer=w388:u8)
                            n130 = Unbundle(w390) -> ("Result"=w389:dbl)  [unwired: 5 out]
                            n131 = Index Array(array=w385, index=w388) -> (element=w386:cluster{string, string})
                          }
                          frame "A4" {
                            n132 = Unbundle(w394) -> ("A4 signál"=w391:enum16{"EMG", "ECG", "EEG", "EDA", "ACC"})  [unwired: 5 out]
                            n133 = To Unsigned Byte Integer(number=w391) -> (unsigned 8bit integer=w395:u8)
                            n134 = Unbundle(w397) -> ("Result"=w396:dbl)  [unwired: 5 out]
                            n135 = Index Array(array=w393, index=w395) -> (element=w392:cluster{string, string})
                          }
                          frame "A5" {
                            n136 = Unbundle(w401) -> ("A5 signál"=w398:enum16{"EMG", "ECG", "EEG", "EDA", "ACC"})  [unwired: 5 out]
                            n137 = Unbundle(w404) -> ("Result"=w403:dbl)  [unwired: 5 out]
                            n138 = To Unsigned Byte Integer(number=w398) -> (unsigned 8bit integer=w402:u8)
                            n139 = Index Array(array=w399, index=w402) -> (element=w400:cluster{string, string})
                          }
                          frame "A6" {
                            n140 = Unbundle(w408) -> ("A6 signál"=w405:enum16{"EMG", "ECG", "EEG", "EDA", "ACC"})  [unwired: 5 out]
                            n141 = To Unsigned Byte Integer(number=w405) -> (unsigned 8bit integer=w409:u8)
                            n142 = Unbundle(w411) -> ("Result"=w410:dbl)  [unwired: 5 out]
                            n143 = Index Array(array=w407, index=w409) -> (element=w406:cluster{string, string})
                          }
                        }
                        "Ylabel and Plot name" <- w323
                        "Zobrazeni typu signalu" <- w323
                        n144 = Rotate 1D Array(1:w350, 2:1 ("n")) -> (0:w352:dbl[])
                        n145 = Rotate 1D Array(1:w347, 2:1 ("n")) -> (0:w348:dbl[])
                        n146 = Replace Array Subset(array=w352, new element=w340) -> (w321:dbl[])  [unwired: 1 in]
                        n147 = Replace Array Subset(array=w348, new element=w346) -> (w326:dbl[])  [unwired: 1 in]
                        n148 = Unbundle(w323) -> (w335:string)  [unwired: 1 out]
                        n149 = Build Array(w340) -> (w339:dbl[])
                        n150 = Reverse 1D Array(array=w326) -> (reversed array=w325:dbl[])
                        n151 = Reverse 1D Array(array=w321) -> (reversed array=w322:dbl[])
                        n152 = Reciprocal(x=w319) -> (1/x=w320:dbl)
                        n153 = Bundle(w322, w325) -> (→"XY graph visual":cluster{dbl[], dbl[]})  [unwired: 1 in]
                        n154 = Bundle By Name("Y"=w321, "dt"=w320) -> (w318:waveform(dbl))  [unwired: 1 in]
                        n155 = TDMS Write(0:w343, 5:"bitalino", 7:w335, 9:w339, 11:w341) -> (4:w342:refnum<k34>, 15:w338:errorcluster)  [unwired: 1 in, 2 out]
                      }
                      frame Error {
                      }
                    }
                    "Consumer" <- w304
                  }
                  n156 = while {
                    tunnel: w249 -> [w271]
                    stop <- w268 stop-if-true
                    # "Update property nodes for every second"
                    n157 = Dequeue Element(queue=w271) -> (element=w269:bool, error out=w270:errorcluster)  [unwired: 2 in, 2 out]
                    n158 = case shown="No Error" w270 {
                      tunnel: w269 -> [w275 _]
                      tunnel: [FALSE TRUE] -> w268
                      frame No Error {
                        # "7."
                        n159 = property on="Ylabel and Plot name" class="Clust (strict)"() -> ("Value"=w278:cluster{string, string})  [unwired: 2 in, 2 out]
                        n160 = Unbundle(w278) -> (w277:string, w276:string)
                        n161 = property on="XY graph visual" class="XYGraph (strict)"() -> ("Plot.Plot Name"=w272:string)  [unwired: 2 in, 2 out]
                        n162 = property on="XY graph visual" class="XYGraph (strict)"() -> ("YScale.NameLbl.Text"=w273:string)  [unwired: 2 in, 2 out]
                        n163 = case shown="True" w275 {
                          tunnel: w273 -> [_ w284]
                          tunnel: w272 -> [_ w280]
                          tunnel: w277 -> [_ w281]
                          tunnel: w276 -> [_ w279]
                          frame False {
                          }
                          frame True {
                            n164 = Not Equal?(x=w284, y=w281) -> (x != y?=w282:bool)
                            n165 = Not Equal?(x=w280, y=w279) -> (x != y?=w283:bool)
                            n166 = case shown="True" w282 {
                              tunnel: w281 -> [_ w286]
                              frame False {
                              }
                              frame True {
                                n167 = property on="XY graph visual" class="XYGraph (strict)"("YScale.NameLbl.Text"=w286) -> ()  [unwired: 2 in, 2 out]
                              }
                            }
                            n168 = case shown="True" w283 {
                              tunnel: w279 -> [_ w285]
                              frame False {
                              }
                              frame True {
                                n169 = property on="XY graph visual" class="XYGraph (strict)"("Plot.Plot Name"=w285) -> ()  [unwired: 2 in, 2 out]
                              }
                            }
                          }
                        }
                      }
                      frame Error {
                      }
                    }
                  }
                  n170 = while {
                    shift-right: [w432] -> w258
                    shift-left: w264 -> [w423]
                    shift-right: [w433] -> w261
                    shift-left: w263 -> [w434]
                    shift-right: [w431] -> w260
                    shift-left: w232 -> [w422]
                    tunnel: w231 -> [w420]
                    i -> [w428]
                    stop <- w427 stop-if-true
                    # "Reading"
                    n171 = case shown="True" w420 {
                      tunnel: [w437 w446] -> w424
                      tunnel: w423 -> [w436 w440]
                      tunnel: w422 -> [w437 w439]
                      tunnel: [w436 w438] -> w421
                      frame False {
                      }
                      frame True {
                        # "5."
                        n172 = call <userlib>:"Digital IO.vi"("DO 4"="DO 4", "DO 3"="DO 3", "DO in"="DO 2", "DO 1"="DO 1") -> ("string"=w445:string)
                        n173 = VISA Write(VISA resource name=w439, write buffer=w445, error in (no error)=w440) -> (VISA resource name out=w446:refnum<visa-resource-name>, error out=w438:errorcluster)  [unwired: 1 out]
                      }
                    }
                    n174 = VISA Read(VISA resource name=w424, byte count=u32 8, error in (no error)=w421) -> (VISA resource name out=w431:refnum<visa-resource-name>, read buffer=w430:string, error out=w435:errorcluster)  [unwired: 1 out]
                    n175 = Enqueue Element(queue=w434, element=w430, error in (no error)=w435) -> (queue out=w433:refnum<queue>, error out=w432:errorcluster)  [unwired: 1 in, 1 out]
                    n176 = Unbundle By Name(w432) -> ("status"=w425:bool)
                    n177 = local read "Sync Stop"() -> (w426:bool)
                    n178 = Compound Arithmetic op=OR(w425, w426) -> (w427:bool)
                    "producer" <- w428
                  }
                  n179 = call <userlib>:"Wait.vi"("error in (no error)"=w258) -> ("error out"=w259:errorcluster)  [unwired: 10 in]
                  n180 = Build Array(u8 0) -> (w266:u8[])
                  n181 = Byte Array To String(unsigned byte array=w266) -> (string=w265:string)
                  n182 = VISA Write(VISA resource name=w260, write buffer=w265, error in (no error)=w259) -> (VISA resource name out=w256:refnum<visa-resource-name>, error out=w257:errorcluster)  [unwired: 1 out]
                  n183 = VISA Close(VISA resource name=w256, error in (no error)=w257) -> (error out=w255:errorcluster)
                  n184 = Release Queue(queue=w248, error in (no error)=w247) -> (error out=w234:errorcluster)  [unwired: 1 in, 2 out]
                  n185 = Release Queue(queue=w261, error in (no error)=w255) -> (error out=w253:errorcluster)  [unwired: 1 in, 2 out]
                  n186 = TDMS Close(8:w234, 11:w233) -> ()  [unwired: 2 out]
                  n187 = Generate User Event(user event=w254, event data cluster=w253) -> ()  [unwired: 2 in, 2 out]
                }
                frame Error {
                  n188 = Generate User Event(user event=w450, event data cluster=w449) -> ()  [unwired: 2 in, 2 out]
                }
              }
            }
            frame "Exit" {
              n189 = flat-sequence {
                frame #0 {
                  n190 = property on="Stop Button" class="Bool"("DisabledEnum"=T3."Enabled" ("Disabled")) -> ()  [unwired: 2 in, 2 out]
                }
                frame #1 {
                  n191 = Stop(stop? (T)=TRUE) -> ()
                }
              }
            }
          }
        }
        frame Error {
        }
      }
    }
    n192 = while {
      shift-right: [w462] -> w29
      shift-left: w25 -> [w465]
      shift-right: [w463] -> w28
      shift-left: w26 -> [w464]
      tunnel: w21 -> [w459]
      tunnel: [w458] -> w18
      stop <- w461 stop-if-true
      # "1."
      # "State Machine"
      n193 = event shown="[3] \"MereniAZpracovaniSwitch\": Value Change" {
        selector: w459 -> [_ _ _ _ _]
        dyn-events: [_ _ _ _ _] -> w458
        timeout: _ -> [_ _ _ _ _]
        tunnel: w465 -> [w472 w476 w488 w493 w498]
        tunnel: w464 -> [w469 w478 w487 w491 w496]
        tunnel: [w466 w479 w482 w490 w495] -> w463
        tunnel: [w473 w477 w484 w492 w497] -> w462
        tunnel: [FALSE TRUE FALSE _ _] -> w461
        event "Cluster.Stop Button": Value Change {
          n194 = event-data() -> ()  [unwired: 1 in, 5 out]
          n195 = Enqueue Element(queue=w472, element=Status."Standby" ("Enum"), error in (no error)=w469) -> (queue out=w473:refnum<queue>, error out=w467:errorcluster)  [unwired: 1 in, 1 out]
          n196 = property on="Sync Stop" class="Bool (strict)"(error in=w467, "Val(Sgnl)"=TRUE) -> (error out=w466:errorcluster)  [unwired: 1 in, 1 out]
        }
        event "Exit Button": Value Change {
          n197 = event-data() -> ()  [unwired: 1 in, 5 out]
          n198 = Enqueue Element(queue=w476, element=Status."Exit" ("Enum"), error in (no error)=w478) -> (queue out=w477:refnum<queue>, error out=w479:errorcluster)  [unwired: 1 in, 1 out]
        }
        event "Cluster.Record Button": Value Change {
          n199 = event-data() -> ()  [unwired: 1 in, 1 out]
          n200 = Enqueue Element(queue=w488, element=Status."Initialize" ("Enum"), error in (no error)=w487) -> (queue out=w485:refnum<queue>, error out=w483:errorcluster)  [unwired: 1 in, 1 out]
          n201 = Enqueue Element(queue=w485, element=Status."Recording" ("Enum"), error in (no error)=w483) -> (queue out=w484:refnum<queue>, error out=w482:errorcluster)  [unwired: 1 in, 1 out]
        }
        event "MereniAZpracovaniSwitch": Value Change {
          n202 = event-data() -> ("OldVal"=w494:bool)  [unwired: 1 in]
          "NewVal" <- w494
          n203 = property on="Cluster" class="Clust"("Visible"=w494) -> ()  [unwired: 2 in, 2 out]
          n204 = Enqueue Element(queue=w493, element=Status."Edit", error in (no error)=w491) -> (queue out=w492:refnum<queue>, error out=w490:errorcluster)  [unwired: 1 in, 1 out]
        }
        event User Event {
          n205 = event-data() -> ()  [unwired: 1 in, 1 out]
          n206 = Enqueue Element(queue=w498, element=Status."Standby" ("Enum"), error in (no error)=w496) -> (queue out=w497:refnum<queue>, error out=w495:errorcluster)  [unwired: 1 in, 1 out]
        }
      }
      n207 = Wait Until Next ms Multiple(millisecond multiple=u32 250) -> ()  [unwired: 1 out]
    }
    n208 = Release Queue(queue=w29, error in (no error)=w28) -> (error out=w19:errorcluster)  [unwired: 1 in, 2 out]
    n209 = Unregister For Events(event registration refnum=w18, error in=w19) -> (error out=w17:errorcluster)
    n210 = Destroy User Event(user event=w16, error in=w17) -> ()  [unwired: 1 out]
  }
